vi "Close Shutter.vi"(8 "error in (no error)":errorcluster, 10 "Shutter to Close":T1=enum."Cy3 (532 nm)", 11 "Uniblitz Shutter in":refnum<class "Uniblitz Shutter.lvclass">) -> (0 "error out":errorcluster, 3 "Uniblitz Shutter out":refnum<class "Uniblitz Shutter.lvclass">)   [LabVIEW 2015, in "Uniblitz Shutter.lvlib" / "Uniblitz Shutter.lvclass"]
uses:
  Uniblitz Shutter.lvclass
  Resources/Type Defs/Excitation.ctl
  Uniblitz Shutter.lvclass/Uniblitz Shutter.ctl
  <vilib>/DAQmx/write.llb/DAQmx Write (Digital Bool 1Line 1Point).vi
  <vilib>/DAQmx/miscellaneous.llb/DAQmx Fill In Error Info.vi
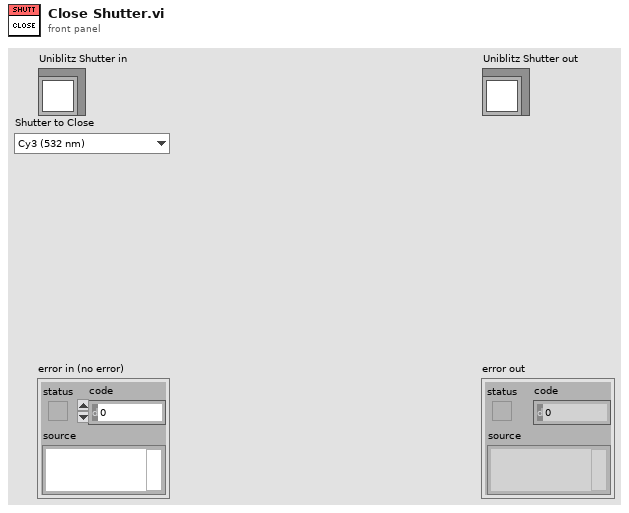
[diagram p1: front panel]
types:
  T1 = typedef "Excitation.ctl" = enum16{"Cy2 (473 nm)", "Cy3 (532 nm)", "Cy5 (639 nm)", "Cy7 (730 nm)", "Cy2/Cy3", "Cy3/Cy5", "Cy3/Cy7", "Cy5/Cy7"}
  T2 = cluster{"Excitation":T1, "DAQmx Channel":refnum<k21>, "Open?":bool}[]
  T3 = cluster{"Excitation":T1, "DAQmx Channel":refnum<k21>, "Open?":bool}
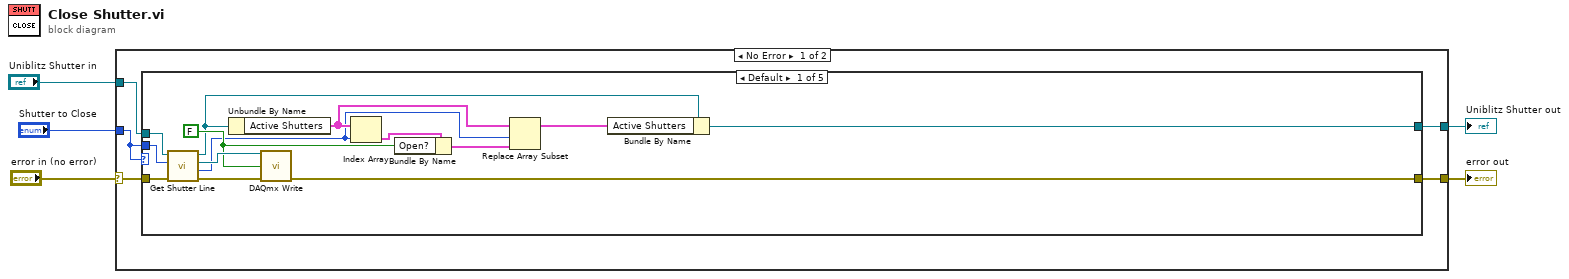
[diagram p0: block diagram]
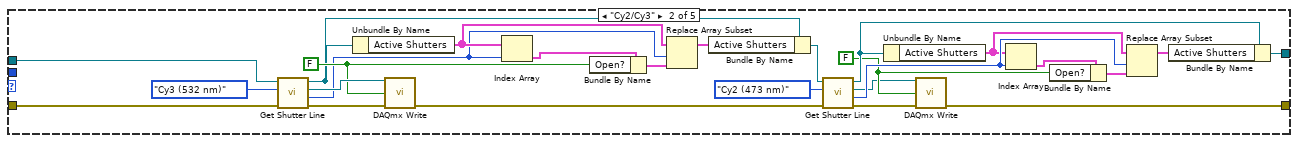
[diagram p2: hidden frame]
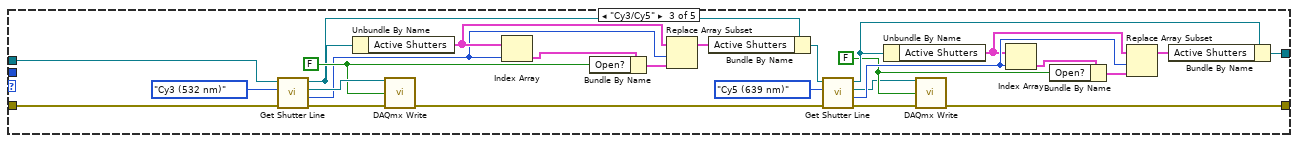
[diagram p3: hidden frame]
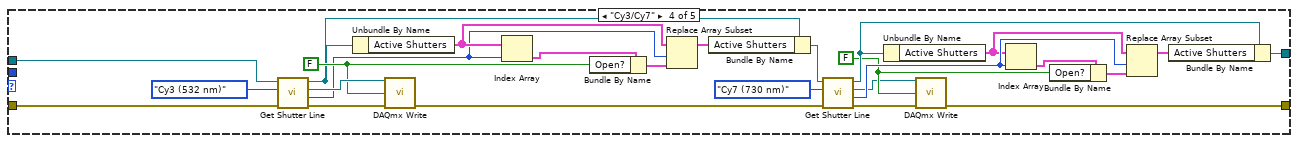
[diagram p4: hidden frame]
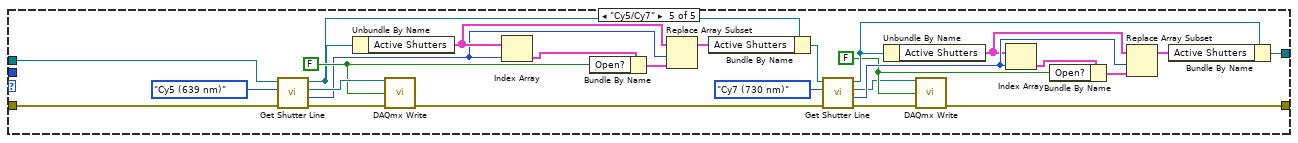
[diagram p5: hidden frame]
diagram:
  n1 = case shown="No Error" "error in (no error)" {
    selector: "error in (no error)" -> [w9 w130]
    tunnel: [w8 w130] -> w5
    tunnel: [w7 w129] -> w4
    tunnel: "Uniblitz Shutter in" -> [w10 w129]
    tunnel: "Shutter to Close" -> [w6 _]
    frame No Error {
      n2 = case shown="Default" w6 {
        tunnel: w10 -> [w24 w50 w76 w102 w128]
        tunnel: w6 -> [w23 _ _ _ _]
        tunnel: w9 -> [w22 w49 w75 w101 w127]
        tunnel: [w19 w28 w54 w80 w106] -> w8
        tunnel: [w11 w27 w53 w79 w105] -> w7
        frame Default {
          w17 = FALSE ("data")
          n3 = call-dynamic "Get Shutter Line.vi"("error in (no error)"=w22, "Shutter"=w23, "Uniblitz Shutter in"=w24) -> ("error out"=w20:errorcluster, "Index"=w14:i32, "DAQmx Channel"=w21:refnum<k21>, "Uniblitz Shutter out"=w12:refnum<class "Uniblitz Shutter.lvclass">)  [unwired: 5 in]
          n4 = Unbundle By Name(w12) -> ("Active Shutters"=w16:T2)
          n5 = call-poly <vilib>:"DAQmx Write.vi"("task/channels in"=w21, "data"=w17, "error in"=w20) -> ("error out"=w19:errorcluster)  [unwired: 10 in, 2 out]
          n6 = Index Array(array=w16, index=w14) -> (element=w18:T3)
          n7 = Bundle By Name(cluster=w18, "Open?"=w17) -> (w15:T3)
          n8 = Replace Array Subset(array=w16, new element=w15, index=w14) -> (w13:T2)
          n9 = Bundle By Name(cluster=w12, "Active Shutters"=w13) -> (w11:refnum<class "Uniblitz Shutter.lvclass">)
        }
        frame "Cy2/Cy3" {
          w34 = FALSE ("data")
          w45 = FALSE ("data")
          n10 = call-dynamic "Get Shutter Line.vi"("error in (no error)"=w49, "Shutter"=Excitation."Cy3 (532 nm)", "Uniblitz Shutter in"=w50) -> ("error out"=w47:errorcluster, "Index"=w42:i32, "DAQmx Channel"=w48:refnum<k21>, "Uniblitz Shutter out"=w40:refnum<class "Uniblitz Shutter.lvclass">)  [unwired: 5 in]
          n11 = Unbundle By Name(w40) -> ("Active Shutters"=w44:T2)
          n12 = call-poly <vilib>:"DAQmx Write.vi"("task/channels in"=w48, "data"=w45, "error in"=w47) -> ("error out"=w29:errorcluster)  [unwired: 10 in, 2 out]
          n13 = Index Array(array=w44, index=w42) -> (element=w46:T3)
          n14 = Bundle By Name(cluster=w46, "Open?"=w45) -> (w43:T3)
          n15 = Replace Array Subset(array=w44, new element=w43, index=w42) -> (w41:T2)
          n16 = Bundle By Name(cluster=w40, "Active Shutters"=w41) -> (w30:refnum<class "Uniblitz Shutter.lvclass">)
          n17 = call-dynamic "Get Shutter Line.vi"("error in (no error)"=w29, "Shutter"=Excitation."Cy2 (473 nm)", "Uniblitz Shutter in"=w30) -> ("error out"=w32:errorcluster, "Index"=w37:i32, "DAQmx Channel"=w31:refnum<k21>, "Uniblitz Shutter out"=w39:refnum<class "Uniblitz Shutter.lvclass">)  [unwired: 5 in]
          n18 = Unbundle By Name(w39) -> ("Active Shutters"=w35:T2)
          n19 = call-poly <vilib>:"DAQmx Write.vi"("task/channels in"=w31, "data"=w34, "error in"=w32) -> ("error out"=w28:errorcluster)  [unwired: 10 in, 2 out]
          n20 = Index Array(array=w35, index=w37) -> (element=w33:T3)
          n21 = Bundle By Name(cluster=w33, "Open?"=w34) -> (w36:T3)
          n22 = Replace Array Subset(array=w35, new element=w36, index=w37) -> (w38:T2)
          n23 = Bundle By Name(cluster=w39, "Active Shutters"=w38) -> (w27:refnum<class "Uniblitz Shutter.lvclass">)
        }
        frame "Cy3/Cy5" {
          w60 = FALSE ("data")
          w71 = FALSE ("data")
          n24 = call-dynamic "Get Shutter Line.vi"("error in (no error)"=w75, "Shutter"=Excitation."Cy3 (532 nm)", "Uniblitz Shutter in"=w76) -> ("error out"=w73:errorcluster, "Index"=w68:i32, "DAQmx Channel"=w74:refnum<k21>, "Uniblitz Shutter out"=w66:refnum<class "Uniblitz Shutter.lvclass">)  [unwired: 5 in]
          n25 = Unbundle By Name(w66) -> ("Active Shutters"=w70:T2)
          n26 = call-poly <vilib>:"DAQmx Write.vi"("task/channels in"=w74, "data"=w71, "error in"=w73) -> ("error out"=w55:errorcluster)  [unwired: 10 in, 2 out]
          n27 = Index Array(array=w70, index=w68) -> (element=w72:T3)
          n28 = Bundle By Name(cluster=w72, "Open?"=w71) -> (w69:T3)
          n29 = Replace Array Subset(array=w70, new element=w69, index=w68) -> (w67:T2)
          n30 = Bundle By Name(cluster=w66, "Active Shutters"=w67) -> (w56:refnum<class "Uniblitz Shutter.lvclass">)
          n31 = call-dynamic "Get Shutter Line.vi"("error in (no error)"=w55, "Shutter"=Excitation."Cy5 (639 nm)", "Uniblitz Shutter in"=w56) -> ("error out"=w58:errorcluster, "Index"=w63:i32, "DAQmx Channel"=w57:refnum<k21>, "Uniblitz Shutter out"=w65:refnum<class "Uniblitz Shutter.lvclass">)  [unwired: 5 in]
          n32 = Unbundle By Name(w65) -> ("Active Shutters"=w61:T2)
          n33 = call-poly <vilib>:"DAQmx Write.vi"("task/channels in"=w57, "data"=w60, "error in"=w58) -> ("error out"=w54:errorcluster)  [unwired: 10 in, 2 out]
          n34 = Index Array(array=w61, index=w63) -> (element=w59:T3)
          n35 = Bundle By Name(cluster=w59, "Open?"=w60) -> (w62:T3)
          n36 = Replace Array Subset(array=w61, new element=w62, index=w63) -> (w64:T2)
          n37 = Bundle By Name(cluster=w65, "Active Shutters"=w64) -> (w53:refnum<class "Uniblitz Shutter.lvclass">)
        }
        frame "Cy3/Cy7" {
          w86 = FALSE ("data")
          w97 = FALSE ("data")
          n38 = call-dynamic "Get Shutter Line.vi"("error in (no error)"=w101, "Shutter"=Excitation."Cy3 (532 nm)", "Uniblitz Shutter in"=w102) -> ("error out"=w99:errorcluster, "Index"=w94:i32, "DAQmx Channel"=w100:refnum<k21>, "Uniblitz Shutter out"=w92:refnum<class "Uniblitz Shutter.lvclass">)  [unwired: 5 in]
          n39 = Unbundle By Name(w92) -> ("Active Shutters"=w96:T2)
          n40 = call-poly <vilib>:"DAQmx Write.vi"("task/channels in"=w100, "data"=w97, "error in"=w99) -> ("error out"=w81:errorcluster)  [unwired: 10 in, 2 out]
          n41 = Index Array(array=w96, index=w94) -> (element=w98:T3)
          n42 = Bundle By Name(cluster=w98, "Open?"=w97) -> (w95:T3)
          n43 = Replace Array Subset(array=w96, new element=w95, index=w94) -> (w93:T2)
          n44 = Bundle By Name(cluster=w92, "Active Shutters"=w93) -> (w82:refnum<class "Uniblitz Shutter.lvclass">)
          n45 = call-dynamic "Get Shutter Line.vi"("error in (no error)"=w81, "Shutter"=Excitation."Cy7 (730 nm)", "Uniblitz Shutter in"=w82) -> ("error out"=w84:errorcluster, "Index"=w89:i32, "DAQmx Channel"=w83:refnum<k21>, "Uniblitz Shutter out"=w91:refnum<class "Uniblitz Shutter.lvclass">)  [unwired: 5 in]
          n46 = Unbundle By Name(w91) -> ("Active Shutters"=w87:T2)
          n47 = call-poly <vilib>:"DAQmx Write.vi"("task/channels in"=w83, "data"=w86, "error in"=w84) -> ("error out"=w80:errorcluster)  [unwired: 10 in, 2 out]
          n48 = Index Array(array=w87, index=w89) -> (element=w85:T3)
          n49 = Bundle By Name(cluster=w85, "Open?"=w86) -> (w88:T3)
          n50 = Replace Array Subset(array=w87, new element=w88, index=w89) -> (w90:T2)
          n51 = Bundle By Name(cluster=w91, "Active Shutters"=w90) -> (w79:refnum<class "Uniblitz Shutter.lvclass">)
        }
        frame "Cy5/Cy7" {
          w112 = FALSE ("data")
          w123 = FALSE ("data")
          n52 = call-dynamic "Get Shutter Line.vi"("error in (no error)"=w127, "Shutter"=Excitation."Cy5 (639 nm)", "Uniblitz Shutter in"=w128) -> ("error out"=w125:errorcluster, "Index"=w120:i32, "DAQmx Channel"=w126:refnum<k21>, "Uniblitz Shutter out"=w118:refnum<class "Uniblitz Shutter.lvclass">)  [unwired: 5 in]
          n53 = Unbundle By Name(w118) -> ("Active Shutters"=w122:T2)
          n54 = call-poly <vilib>:"DAQmx Write.vi"("task/channels in"=w126, "data"=w123, "error in"=w125) -> ("error out"=w107:errorcluster)  [unwired: 10 in, 2 out]
          n55 = Index Array(array=w122, index=w120) -> (element=w124:T3)
          n56 = Bundle By Name(cluster=w124, "Open?"=w123) -> (w121:T3)
          n57 = Replace Array Subset(array=w122, new element=w121, index=w120) -> (w119:T2)
          n58 = Bundle By Name(cluster=w118, "Active Shutters"=w119) -> (w108:refnum<class "Uniblitz Shutter.lvclass">)
          n59 = call-dynamic "Get Shutter Line.vi"("error in (no error)"=w107, "Shutter"=Excitation."Cy7 (730 nm)", "Uniblitz Shutter in"=w108) -> ("error out"=w110:errorcluster, "Index"=w115:i32, "DAQmx Channel"=w109:refnum<k21>, "Uniblitz Shutter out"=w117:refnum<class "Uniblitz Shutter.lvclass">)  [unwired: 5 in]
          n60 = Unbundle By Name(w117) -> ("Active Shutters"=w113:T2)
          n61 = call-poly <vilib>:"DAQmx Write.vi"("task/channels in"=w109, "data"=w112, "error in"=w110) -> ("error out"=w106:errorcluster)  [unwired: 10 in, 2 out]
          n62 = Index Array(array=w113, index=w115) -> (element=w111:T3)
          n63 = Bundle By Name(cluster=w111, "Open?"=w112) -> (w114:T3)
          n64 = Replace Array Subset(array=w113, new element=w114, index=w115) -> (w116:T2)
          n65 = Bundle By Name(cluster=w117, "Active Shutters"=w116) -> (w105:refnum<class "Uniblitz Shutter.lvclass">)
        }
      }
    }
    frame Error {
    }
  }
  "error out" <- w5
  "Uniblitz Shutter out" <- w4
